vi "Save_MES_LogPASS.vi"() -> ()   [LabVIEW 2018]
uses:
  Subvi/Global.vi
  <vilib>/Utility/config.llb/Read Key (String).vi
  <vilib>/Utility/config.llb/NI_LVConfig.lvlib
panel:
  out "路径":path
  out "数组":path[](array[path])
  in  "所有测试数据":string[][](array[string])=[["SN", "NA", "NA", "NA", "NA", "NA", "NA", "NA", "NA", ""], ["AC(mA)", "54", "42", "654", "354", "34", "543", "25", "45", ""], ["IR(Mohm)", "54", "42", "654", "354", "34", "543", "25", "45", ""], ["Result", "PASS", "FAIL", "PASS", "FAIL", "PASS", "FAIL", "FAIL", "FAIL", ""], ["", "", "", "", "", "", "", "", "", "NA"]]
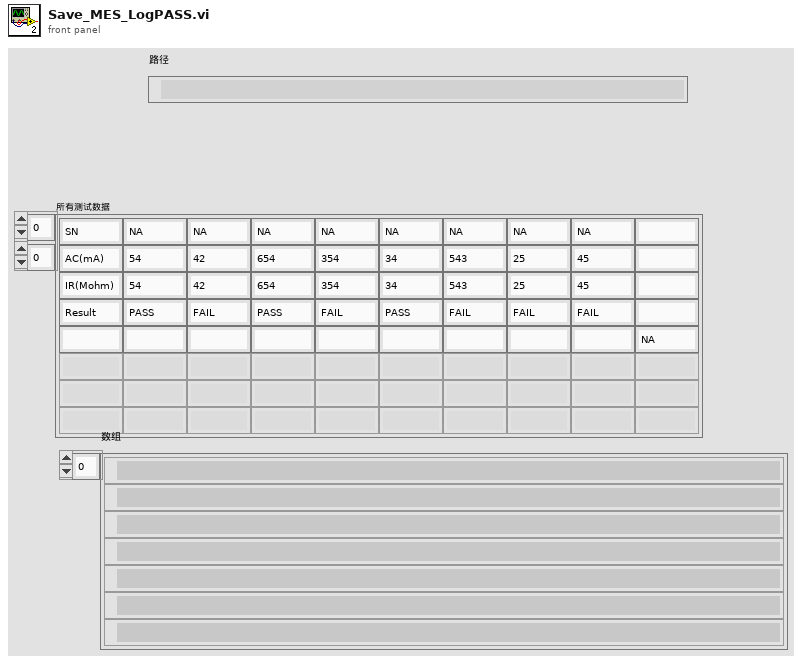
[diagram p1: front panel]
types:
  T1 = typedef "NI_LVConfig.lvlib/Config Data RefNum.ctl" = refnum<k1>
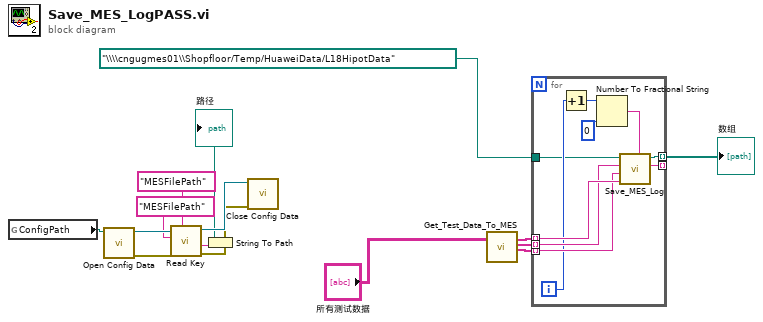
[diagram p0: block diagram]
diagram:
  n1 = global read "Global.vi" "ConfigPath"() -> (w14:path)
  n2 = call <vilib>:"Open Config Data.vi"("configuration file path"=w14) -> ("error out"=w8:errorcluster, "refnum"=w12:T1)  [unwired: 8 in, 1 out]
  n3 = call-poly <vilib>:"Read Key.vi"("section"="MESFilePath", "error in (no error)"=w8, "key"="MESFilePath", "refnum"=w12) -> ("error out"=w9:errorcluster, "value"=w15:string, "refnum out"=w13:T1)  [unwired: 4 in, 1 out]
  n4 = String To Path(string=w15) -> (path=→"路径":path)
  n5 = call <vilib>:"Close Config Data.vi"("error in (no error)"=w9, "refnum"=w13) -> ()  [unwired: 8 in, 2 out]
  n6 = call "Get_Test_Data_To_MES.vi"("所有测试数据"="所有测试数据") -> ("数组"=w5:string[], "SN"=w7:string[], "RESULT"=w6:string[])  [unwired: 16 in]
  n7 = for {
    tunnel: w5 -> [w25] mode=indexing
    tunnel: [w24] -> w2 mode=indexing
    tunnel: w6 -> [w23] mode=indexing
    tunnel: w7 -> [w22] mode=indexing
    tunnel: [w21] -> _ mode=indexing
    tunnel: path "\\\\cngugmes01\\Shopfloor/Temp/HuaweiData/L18HipotData" -> [w16]
    i -> [w19]
    n8 = Increment(x=w19) -> (x+1=w18:i32)
    n9 = Number To Fractional String(number=w18, precision (6)=i16 0 ("精度(6)")) -> (F-format string=w17:string)  [unwired: 2 in]
    n10 = call "Save_MES_Log.vi"("XML File Path"=w16, "SerialNumber"=w22, "StatusCode"=w23, "XML Input"=w25, "CELL"=w17) -> ("XML File Path(duplicate)"=w24:path, "XML String"=w21:string)  [unwired: 3 in]
  }
  "数组" <- w2
